vi "Pellet.Reader.vi"   [LabVIEW 2015]
uses:
  <vilib>/NXT/LegoClasses/BrickReference/BrickReference.lvclass
  <vilib>/NXT/Subs/LVHSConnector.ctl
  <vilib>/NXT/NXTIO Xnodes/NXTIOXNode/NXTIO.xnode
  <vilib>/NXT/NXTIO Xnodes/NXTIONodeSubVIs/LEGOMoveAllMotors.vi
  <vilib>/NXT/Dual Mode Library/Sensors/EV3_Color_Color.vi
  <vilib>/NXT/Dual Mode Library/Sensors/Touch_Pressed.vi
  <vilib>/NXT/Dual Mode Library/Display/drawText.vi
types:
  T1 = typedef "ColorSensorColors.ctl" = enum16{"No Color", "Black", "Blue", "Green", "Yellow", "Red", "White", "Brown"}
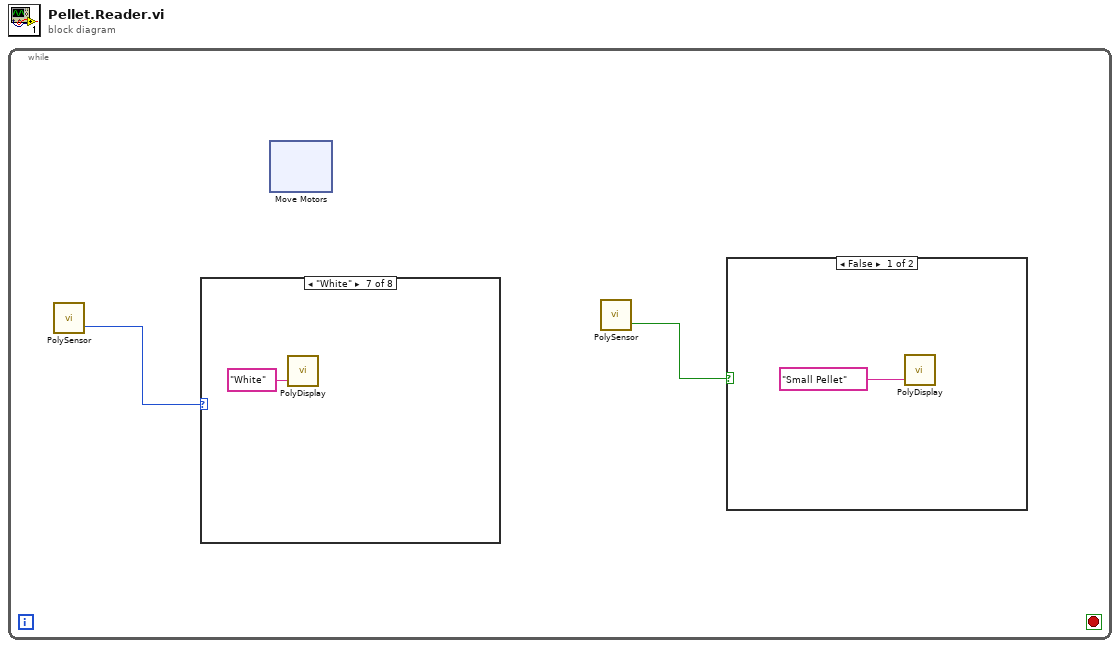
[diagram p0: block diagram]
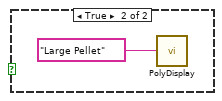
[diagram p2: hidden frame]
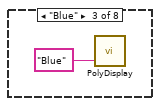
[diagram p5: hidden frame]
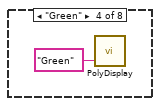
[diagram p6: hidden frame]
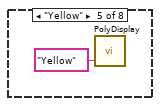
[diagram p7: hidden frame]
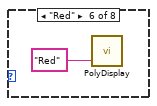
[diagram p8: hidden frame]
diagram:
  n1 = while {
    stop <- _ stop-if-true
    n2 = call-poly <vilib>:"PolySensor.vi"() -> ("Detected Color"=w2:T1)  [unwired: 3 in, 1 out]
    n3 = case shown="\"White\"" w2 {
      frame "No Color", Default {
      }
      frame "Black" {
      }
      frame "Blue" {
        n4 = call-poly <vilib>:"PolyDisplay.vi"("Text"="Blue") -> ()  [unwired: 3 in, 1 out]
      }
      frame "Green" {
        n5 = call-poly <vilib>:"PolyDisplay.vi"("Text"="Green") -> ()  [unwired: 3 in, 1 out]
      }
      frame "Yellow" {
        n6 = call-poly <vilib>:"PolyDisplay.vi"("Text"="Yellow") -> ()  [unwired: 3 in, 1 out]
      }
      frame "Red" {
        n7 = call-poly <vilib>:"PolyDisplay.vi"("Text"="Red") -> ()  [unwired: 3 in, 1 out]
      }
      frame "White" {
        n8 = call-poly <vilib>:"PolyDisplay.vi"("Text"="White") -> ()  [unwired: 3 in, 1 out]
      }
      frame "Brown" {
      }
    }
    n9 = xnode "Move Motors"() -> ()  [unwired: 3 in, 1 out]
    n10 = call-poly <vilib>:"PolySensor.vi"() -> ("Yes / No"=w1:bool)  [unwired: 3 in, 1 out]
    n11 = case shown="False" w1 {
      frame False {
        n12 = call-poly <vilib>:"PolyDisplay.vi"("Text"="Small Pellet") -> ()  [unwired: 3 in, 1 out]
      }
      frame True {
        n13 = call-poly <vilib>:"PolyDisplay.vi"("Text"="Large Pellet") -> ()  [unwired: 3 in, 1 out]
      }
    }
  }
